vi "Update Pin Map for Sequence.vi"(8 "error in":errorcluster, 10 "pin map path":path, 11 "sequence context in":refnum<k7>) -> (0 "error out":errorcluster)   [LabVIEW 2020, in "MeasurementLink Pin Map.lvlib"]
doc: "Updates the pin map service with the contents of the file specified by <b>pin map path</b> for the specified TestStand sequence."
uses:
  MeasurementLink Pin Map.lvlib
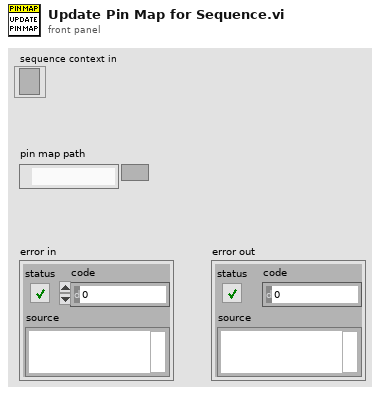
[diagram p1: front panel]
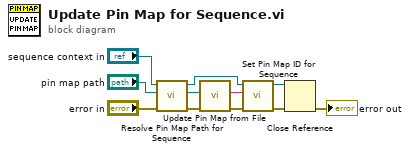
[diagram p0: block diagram]
diagram:
  n1 = call "Resolve Pin Map Path for Sequence.vi"("error in"="error in", "pin map path"="pin map path", "sequence context in"="sequence context in") -> ("error out"=w7:errorcluster, "absolute pin map path"=w2:path, "sequence context out"=w3:refnum<k7>)  [unwired: 6 in]
  n2 = call "Update Pin Map from File.vi"("error in (no error)"=w7, "pin map path"=w2) -> ("error out"=w8:errorcluster, "pin map id"=w1:string)  [unwired: 8 in]
  n3 = call "Set Pin Map ID for Sequence.vi"("error in"=w8, "pin_map_id"=w1, "sequence context in"=w3) -> ("error out"=w11:errorcluster, "sequence context out"=w5:refnum<k7>)  [unwired: 7 in]
  n4 = Close Reference(reference=w5, error in (no error)=w11) -> (error out=→"error out":errorcluster)
